vi "ConstrFinalize.vi"() -> ()   [LabVIEW 2015]
uses:
  GlobalPath.vi
  GlobalData.vi
  GlobalVi.vi
panel:
  in  "ptfe 10":bool caption="Position the panel on the testing table"
  out "PanelName":string
  in  "ptfe 9":bool caption="Move the panel away from the construction table"
  in  "DONE ALL?":bool
  in  "ptfe 5":bool caption="Lift the machine with the panel"
  in  "ptfe 4":bool caption="Switch on the vacuum on the machine"
  in  "ptfe 3":bool caption="Lower the machine on the panel making sure the sucking cups are on the external part of the panel"
  in  "ptfe 2":bool caption="Move the rotating machine on top of the panel"
  # "1. Contruction Finalization"
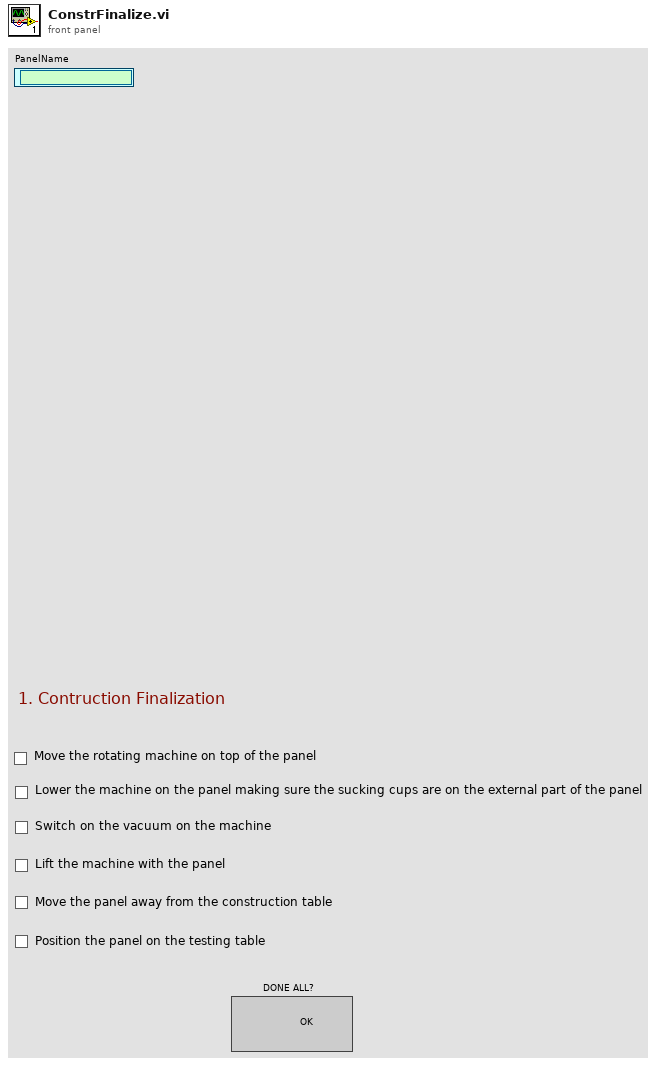
[diagram p1: front panel]
types:
  T1 = enum16{"open", "replace", "create", "open or create", "replace or create", "replace or create with confirmation"}
  T2 = enum32{"Bad", "Idle", "Run top level", "Running"}
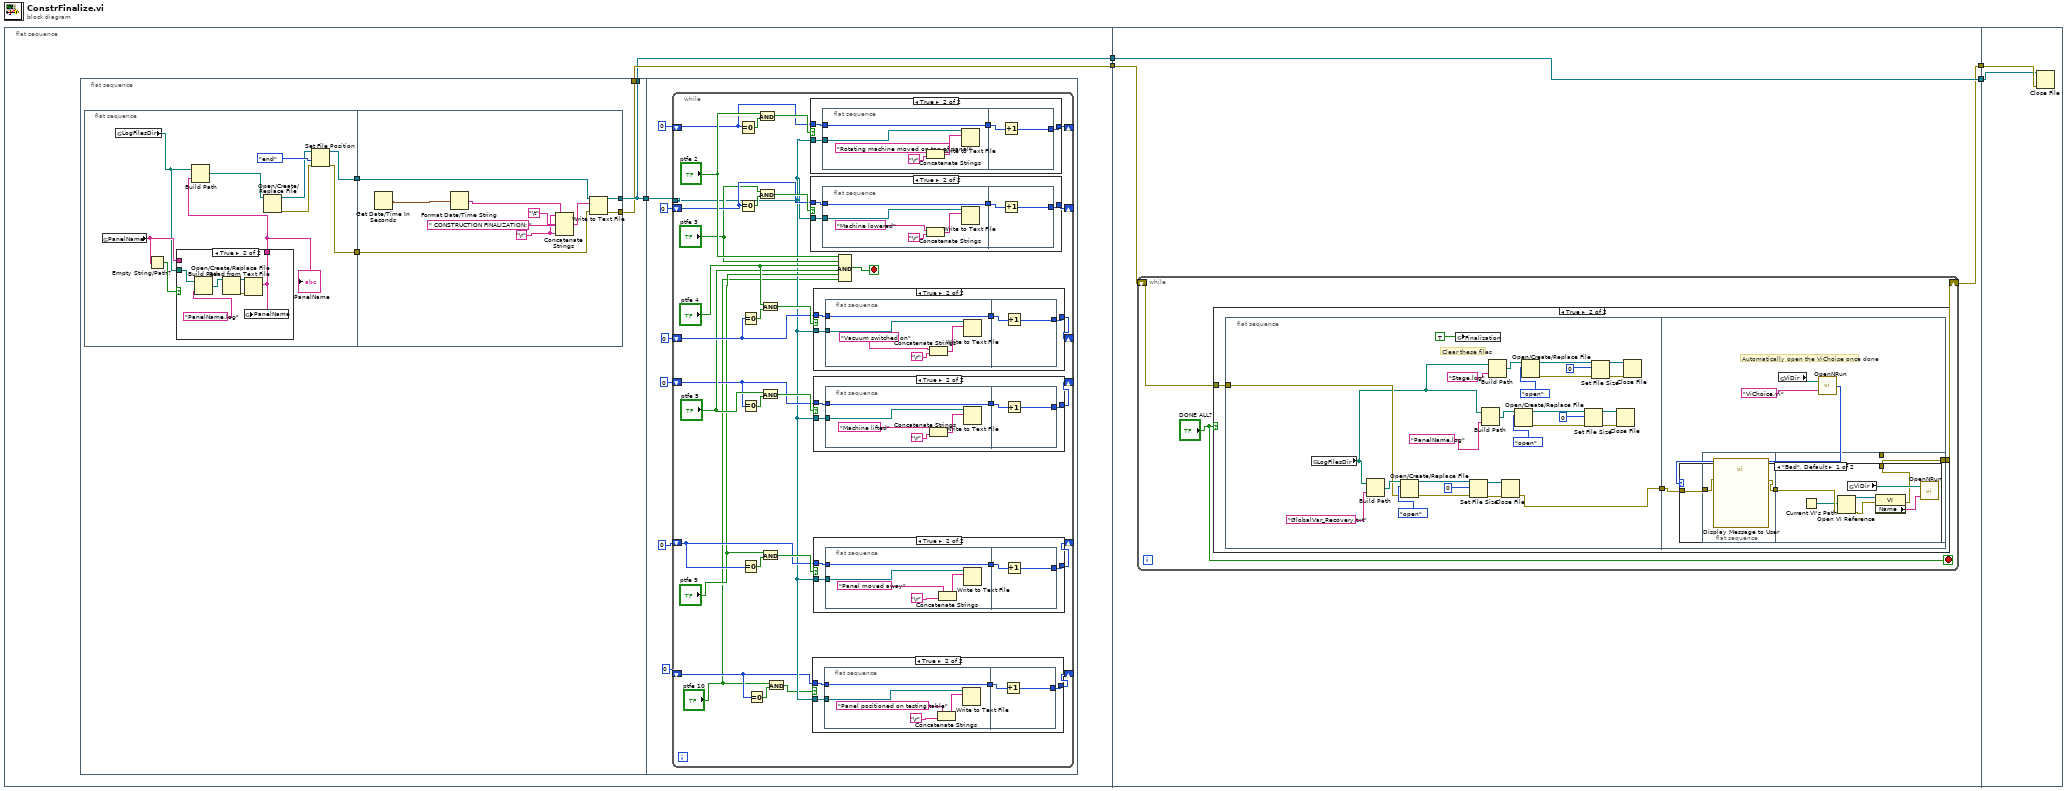
[diagram p0: block diagram]
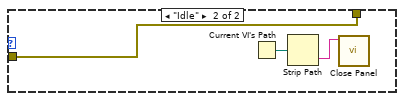
[diagram p10: hidden frame]
diagram:
  n1 = flat-sequence {
    tunnel: [w6] -> w3
    tunnel: [w5] -> w2
    tunnel: [w151] -> w4
    tunnel: w3 -> [w150]
    tunnel: w2 -> [w152]
    tunnel: [w152] -> w1
    tunnel: w4 -> [w209]
    tunnel: w1 -> [w208]
    frame #0 {
      n2 = flat-sequence {
        tunnel: [w10] -> w7
        tunnel: [w10] -> w5
        tunnel: [w9] -> w6
        tunnel: w7 -> [w45]
        frame #0 {
          n3 = flat-sequence {
            tunnel: [w16] -> w11
            tunnel: [w18] -> w8
            tunnel: w11 -> [w34]
            tunnel: [w33] -> w10
            tunnel: [w32] -> w9
            tunnel: w8 -> [w31]
            frame #0 {
              n4 = global read "GlobalData.vi" "PanelName"() -> (w15:string)
              n5 = global read "GlobalPath.vi" "LogFilesDir"() -> (w12:path)
              n6 = Empty String/Path?(string/path=w15) -> (empty?=w14:bool)
              n7 = case shown="True" w14 {
                tunnel: w12 -> [_ w28]
                tunnel: [w22 w23] -> w13
                tunnel: w15 -> [w22 _]
                frame False {
                }
                frame True {
                  n8 = Build Path(base path=w28, name or relative path="PanelName.log") -> (appended path=w27:path)
                  n9 = Open/Create/Replace File(file path (use dialog)=w27) -> (refnum out=w24:refnum<file>, error out=w25:errorcluster)  [unwired: 5 in, 1 out]
                  n10 = Read from Text File(file (use dialog)=w24, error in=w25) -> (text=w23:string)  [unwired: 2 in, 3 out]
                  n11 = global write "GlobalData.vi" "PanelName"(w23) -> ()
                }
              }
              "PanelName" <- w13
              n12 = Build Path(base path=w12, name or relative path=w13) -> (appended path=w21:path)
              n13 = Open/Create/Replace File(file path (use dialog)=w21) -> (refnum out=w17:refnum<file>, error out=w19:errorcluster)  [unwired: 5 in, 1 out]
              n14 = Set File Position(refnum=w17, from (0:start)=enum16{"start", "end", "current"}."end", error in=w19) -> (refnum out=w16:refnum<file>, error out=w18:errorcluster)  [unwired: 1 in]
            }
            frame #1 {
              w29 = "\r"
              n15 = Get Date/Time In Seconds() -> (seconds since 1Jan1904=w30:timestamp)
              n16 = Format Date/Time String(seconds (now)=w30) -> (date/time string=w36:string)  [unwired: 2 in]
              n17 = Concatenate Strings(w29, w36, "\t", " CONSTRUCTION FINALIZATION: ", w29) -> (w35:string)
              n18 = Write to Text File(file (use dialog)=w34, text=w35, error in=w31) -> (refnum out=w33:refnum<file>, error out=w32:errorcluster)  [unwired: 1 in, 1 out]
            }
          }
        }
        frame #1 {
          n19 = while {
            tunnel: w45 -> [w50]
            shift-right: [w72] -> _
            shift-left: 0 -> [w73]
            shift-right: [w68] -> _
            shift-left: 0 -> [w69]
            shift-right: [w62] -> _
            shift-left: 0 -> [w64]
            shift-right: [w57] -> _
            shift-left: 0 -> [w58]
            shift-right: [w53] -> _
            shift-left: 0 -> [w54]
            shift-right: [w49] -> _
            shift-left: 0 -> [w47]
            stop <- w77 stop-if-true
            n20 = Equal To 0?(x=w73) -> (x = 0?=w76:bool)
            n21 = Equal To 0?(x=w69) -> (x = 0?=w71:bool)
            n22 = Equal To 0?(x=w64) -> (x = 0?=w66:bool)
            n23 = Equal To 0?(x=w58) -> (x = 0?=w61:bool)
            n24 = Equal To 0?(x=w54) -> (x = 0?=w56:bool)
            n25 = Equal To 0?(x=w47) -> (x = 0?=w51:bool)
            n26 = And(x="ptfe 2", y=w76) -> (x .and. y?=w75:bool)
            n27 = And(x="ptfe 3", y=w71) -> (x .and. y?=w70:bool)
            n28 = And(x="ptfe 4", y=w66) -> (x .and. y?=w65:bool)
            n29 = And(x="ptfe 5", y=w61) -> (x .and. y?=w60:bool)
            n30 = And(x="ptfe 9", y=w56) -> (x .and. y?=w55:bool)
            n31 = And(x="ptfe 10", y=w51) -> (x .and. y?=w48:bool)
            n32 = case shown="True" w75 {
              tunnel: w50 -> [_ w142]
              tunnel: w73 -> [w138 w140]
              tunnel: [w138 w139] -> w72
              frame False {
              }
              frame True {
                n33 = flat-sequence {
                  tunnel: w142 -> [w145]
                  tunnel: [w144] -> w141
                  tunnel: w140 -> [w144]
                  tunnel: w141 -> [w149]
                  tunnel: [w148] -> w139
                  frame #0 {
                    n34 = Concatenate Strings("Rotating machine moved on top of panel", "\r") -> (w147:string)
                    n35 = Write to Text File(file (use dialog)=w145, text=w147) -> ()  [unwired: 2 in, 3 out]
                  }
                  frame #1 {
                    n36 = Increment(x=w149) -> (x+1=w148:i32)
                  }
                }
              }
            }
            n37 = case shown="True" w70 {
              tunnel: w50 -> [_ w130]
              tunnel: w69 -> [w126 w128]
              tunnel: [w126 w127] -> w68
              frame False {
              }
              frame True {
                n38 = flat-sequence {
                  tunnel: w130 -> [w133]
                  tunnel: [w132] -> w129
                  tunnel: w128 -> [w132]
                  tunnel: w129 -> [w137]
                  tunnel: [w136] -> w127
                  frame #0 {
                    n39 = Concatenate Strings("Machine lowered", "\r") -> (w135:string)
                    n40 = Write to Text File(file (use dialog)=w133, text=w135) -> ()  [unwired: 2 in, 3 out]
                  }
                  frame #1 {
                    n41 = Increment(x=w137) -> (x+1=w136:i32)
                  }
                }
              }
            }
            n42 = case shown="True" w48 {
              tunnel: w50 -> [_ w82]
              tunnel: w47 -> [w78 w80]
              tunnel: [w78 w79] -> w49
              frame False {
              }
              frame True {
                n43 = flat-sequence {
                  tunnel: w82 -> [w85]
                  tunnel: [w84] -> w81
                  tunnel: w80 -> [w84]
                  tunnel: w81 -> [w89]
                  tunnel: [w88] -> w79
                  frame #0 {
                    n44 = Concatenate Strings("Panel positioned on testing table", "\r") -> (w87:string)
                    n45 = Write to Text File(file (use dialog)=w85, text=w87) -> ()  [unwired: 2 in, 3 out]
                  }
                  frame #1 {
                    n46 = Increment(x=w89) -> (x+1=w88:i32)
                  }
                }
              }
            }
            n47 = case shown="True" w65 {
              tunnel: w50 -> [_ w118]
              tunnel: w64 -> [w114 w116]
              tunnel: [w114 w115] -> w62
              frame False {
              }
              frame True {
                n48 = flat-sequence {
                  tunnel: w118 -> [w121]
                  tunnel: [w120] -> w117
                  tunnel: w116 -> [w120]
                  tunnel: w117 -> [w125]
                  tunnel: [w124] -> w115
                  frame #0 {
                    n49 = Concatenate Strings("Vacuum switched on", "\r") -> (w123:string)
                    n50 = Write to Text File(file (use dialog)=w121, text=w123) -> ()  [unwired: 2 in, 3 out]
                  }
                  frame #1 {
                    n51 = Increment(x=w125) -> (x+1=w124:i32)
                  }
                }
              }
            }
            n52 = case shown="True" w60 {
              tunnel: w50 -> [_ w106]
              tunnel: w58 -> [w102 w104]
              tunnel: [w102 w103] -> w57
              frame False {
              }
              frame True {
                n53 = flat-sequence {
                  tunnel: w106 -> [w109]
                  tunnel: [w108] -> w105
                  tunnel: w104 -> [w108]
                  tunnel: w105 -> [w113]
                  tunnel: [w112] -> w103
                  frame #0 {
                    n54 = Concatenate Strings("Machine lifted", "\r") -> (w111:string)
                    n55 = Write to Text File(file (use dialog)=w109, text=w111) -> ()  [unwired: 2 in, 3 out]
                  }
                  frame #1 {
                    n56 = Increment(x=w113) -> (x+1=w112:i32)
                  }
                }
              }
            }
            n57 = case shown="True" w55 {
              tunnel: w50 -> [_ w94]
              tunnel: w54 -> [w90 w92]
              tunnel: [w90 w91] -> w53
              frame False {
              }
              frame True {
                n58 = flat-sequence {
                  tunnel: w94 -> [w97]
                  tunnel: [w96] -> w93
                  tunnel: w92 -> [w96]
                  tunnel: w93 -> [w101]
                  tunnel: [w100] -> w91
                  frame #0 {
                    n59 = Concatenate Strings("Panel moved away", "\r") -> (w99:string)
                    n60 = Write to Text File(file (use dialog)=w97, text=w99) -> ()  [unwired: 2 in, 3 out]
                  }
                  frame #1 {
                    n61 = Increment(x=w101) -> (x+1=w100:i32)
                  }
                }
              }
            }
            n62 = Compound Arithmetic op=AND("ptfe 2", "ptfe 3", "ptfe 4", "ptfe 5", "ptfe 9", "ptfe 10") -> (w77:bool)
          }
        }
      }
    }
    frame #1 {
      n63 = while {
        shift-right: [w155] -> w151
        shift-left: w150 -> [w154]
        stop <- "DONE ALL?" stop-if-true
        n64 = case shown="True" "DONE ALL?" {
          tunnel: [w156 w159] -> w155
          tunnel: w154 -> [w156 w158]
          frame False {
          }
          frame True {
            n65 = flat-sequence {
              tunnel: w158 -> [w183]
              tunnel: [w177] -> w157
              tunnel: [w189] -> w159
              tunnel: w157 -> [w188]
              frame #0 {
                # "Clear these files"
                n66 = global read "GlobalPath.vi" "LogFilesDir"() -> (w160:path)
                n67 = Build Path(base path=w160, name or relative path="GlobalVar_Recovery.txt") -> (appended path=w185:path)
                n68 = Open/Create/Replace File(file path (use dialog)=w185, error in=w183, operation (0:open)=T1."open") -> (refnum out=w182:refnum<file>, error out=w181:errorcluster)  [unwired: 3 in, 1 out]
                n69 = global write "GlobalVi.vi" "Finalization"(TRUE) -> ()
                n70 = Set File Size(4:w181, 6:0, 7:w182) -> (0:w179:errorcluster, 3:w178:refnum<file>)
                n71 = Build Path(base path=w160, name or relative path="PanelName.log") -> (appended path=w176:path)
                n72 = Build Path(base path=w160, name or relative path="Stage.log") -> (appended path=w168:path)
                n73 = Close File(refnum=w178, error in=w179) -> (error out=w177:errorcluster)  [unwired: 1 out]
                n74 = Open/Create/Replace File(file path (use dialog)=w176, operation (0:open)=T1."open") -> (refnum out=w174:refnum<file>, error out=w173:errorcluster)  [unwired: 4 in, 1 out]
                n75 = Open/Create/Replace File(file path (use dialog)=w168, operation (0:open)=T1."open") -> (refnum out=w166:refnum<file>, error out=w165:errorcluster)  [unwired: 4 in, 1 out]
                n76 = Set File Size(4:w173, 6:0, 7:w174) -> (0:w171:errorcluster, 3:w170:refnum<file>)
                n77 = Set File Size(4:w165, 6:0, 7:w166) -> (0:w163:errorcluster, 3:w162:refnum<file>)
                n78 = Close File(refnum=w170, error in=w171) -> ()  [unwired: 2 out]
                n79 = Close File(refnum=w162, error in=w163) -> ()  [unwired: 2 out]
              }
              frame #1 {
                # "Automatically open the ViChoise once done"
                n80 = global read "GlobalPath.vi" "ViDir"() -> (w192:path)
                n81 = call "OpenNRun.vi"("VI name"="ViChoice.vi", "ViDirPath"=w192) -> ("Execution:State"=w191:T2)
                n82 = case shown="\"Bad\", Default" w191 {
                  tunnel: [w193 w205] -> w189
                  tunnel: w188 -> [w194 w205]
                  frame "Bad", Default {
                    n83 = flat-sequence {
                      tunnel: w194 -> [w197]
                      tunnel: [w196] -> w195
                      tunnel: w195 -> [w201]
                      tunnel: [w198] -> w193
                      frame #0 {
                        n84 = call "Display Message to User"("error in (no error)"=w197) -> ("error out"=w196:errorcluster)  [unwired: 9 in, 1 out]
                      }
                      frame #1 {
                        n85 = Current VI's Path() -> (path=w199:path)
                        n86 = Open VI Reference(vi path=w199, error in (no error)=w201) -> (vi reference=w204:refnum<vi>, error out=w203:errorcluster)  [unwired: 4 in]
                        n87 = global read "GlobalPath.vi" "ViDir"() -> (w200:path)
                        n88 = property class="VI"(reference=w204, error in=w203) -> (error out=w198:errorcluster, "Name"=w202:string)  [unwired: 1 out]
                        n89 = call "OpenNRun.vi"("VI name"=w202, "ViDirPath"=w200) -> ()  [unwired: 1 out]
                      }
                    }
                  }
                  frame "Idle" {
                    n90 = Current VI's Path() -> (path=w206:path)
                    n91 = Strip Path(path=w206) -> (name=w207:string)  [unwired: 1 out]
                    n92 = call <vilib>:"Close Panel.vi"("VI name"=w207) -> ()  [unwired: 10 in, 1 out]
                  }
                }
              }
            }
          }
        }
      }
    }
    frame #2 {
      n93 = Close File(refnum=w208, error in=w209) -> ()  [unwired: 2 out]
    }
  }
